vi "Inicialización DACs.vi"(7 "Espera acceso USB":u32, 8 "error in":errorcluster, 11 "ftHandle_in":u32) -> (0 "error out":errorcluster, 3 "ftHandle_out":u32)   [LabVIEW 2009]
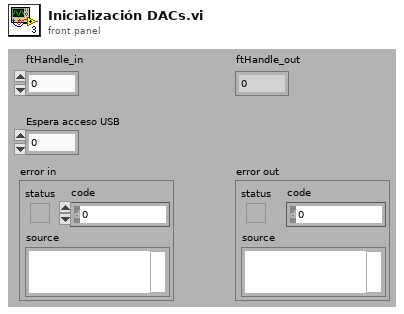
[diagram p1: front panel]
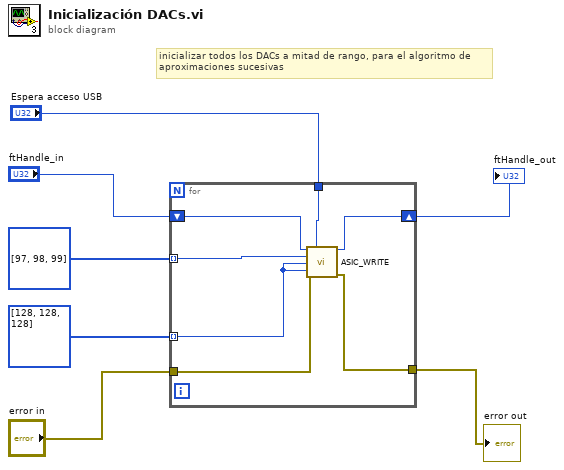
[diagram p0: block diagram]
diagram:
  # "inicializar todos los DACs a mitad de rango, para el algoritmo de aproximaciones sucesivas"
  n1 = for {
    shift-right: [w13] -> w2
    shift-left: "ftHandle_in" -> [w14]
    tunnel: u8[] [97, 98, 99] -> [w12] mode=indexing
    tunnel: u8[] [128, 128, 128] -> [w11] mode=indexing
    tunnel: "error in" -> [w10]
    tunnel: [w9] -> w3
    tunnel: "Espera acceso USB" -> [w8]
    n2 = call "ASIC_WRITE.vi"("ftHandle_in"=w14, "Espera acceso USB"=w8, "Direccion Registro Asic"=w12, "Byte Alto"=w11, "Byte Bajo"=w11, "error in"=w10) -> ("ftHandle_out"=w13:u32, "error out"=w9:errorcluster)  [unwired: 8 in]
  }
  "error out" <- w3
  "ftHandle_out" <- w2
